vi "Select ini file.vi"(7 "error in":errorcluster) -> (0 "error out":errorcluster, 1 "Name":string)   [LabVIEW 2015]
uses:
  New Instance.ctl
  Instance.ctl
  Calibration and Function folders.ctl
  file/file action.ctl
  calibration/Shared Data/share data command.ctl
panel:
  in  "Delete Instance":bool
  in  "Device control":T1 {"Device" items=["Dev6", "Dev10", "Dev11"]}
  in  "Select":bool[](array[boolean])
  out "Instances":T2[](array[typedef])
  in  "New ProCoDA":T3
  in  "OK Button":bool
  # "Currently in use"
  # "Name of this instance"
  # "Method file name"
  # "Name of DAQ"
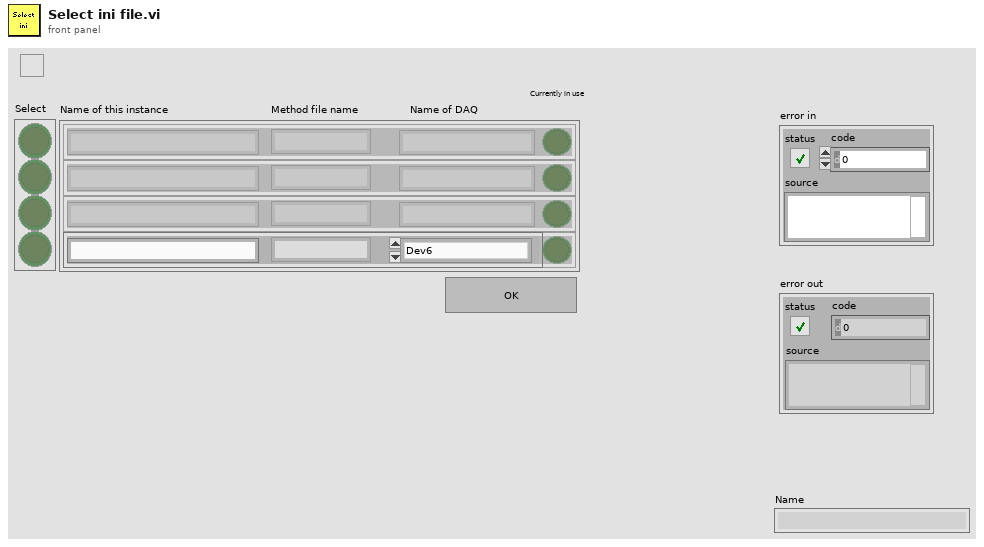
[diagram p1: front panel]
types:
  T1 = cluster{"Name":string, "File Name":string, "Device":u16}
  T2 = typedef "Instance.ctl" = cluster{"Name":string, "Device Name":string, "Running":bool, "File Name":string}
  T3 = typedef "New Instance.ctl" = bool
  T4 = typedef "Calibration and Function folders.ctl" = enum16{"Sensors", "Functions", "Config File", "PublicAppFolder", "New ini File", "Set Config File", "Delete ini File"}
  T5 = typedef "share data command.ctl" = enum16{"Initialize from ini", "Update ini", "Write data", "Read data", "List my data", "List shared data", "Close"}
  T6 = typedef "file action.ctl" = enum16{"Save", "Open"}
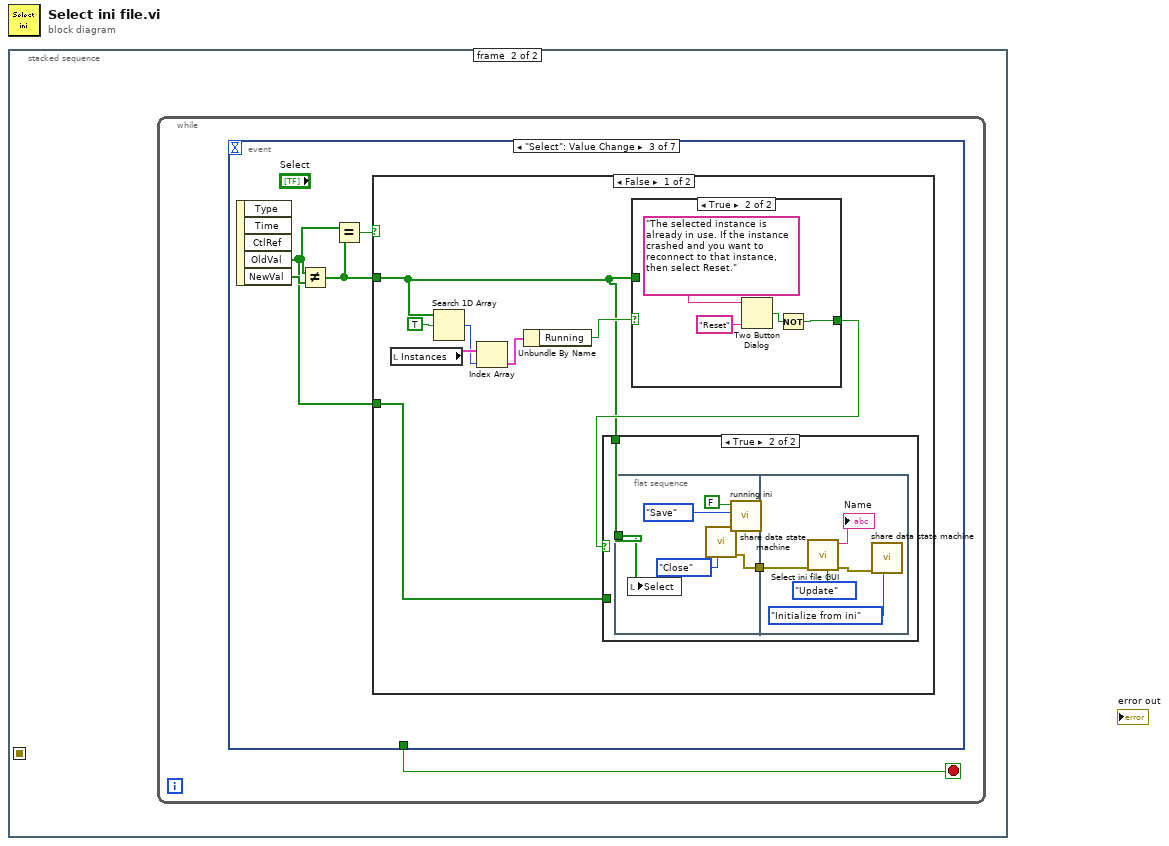
[diagram p0: block diagram]
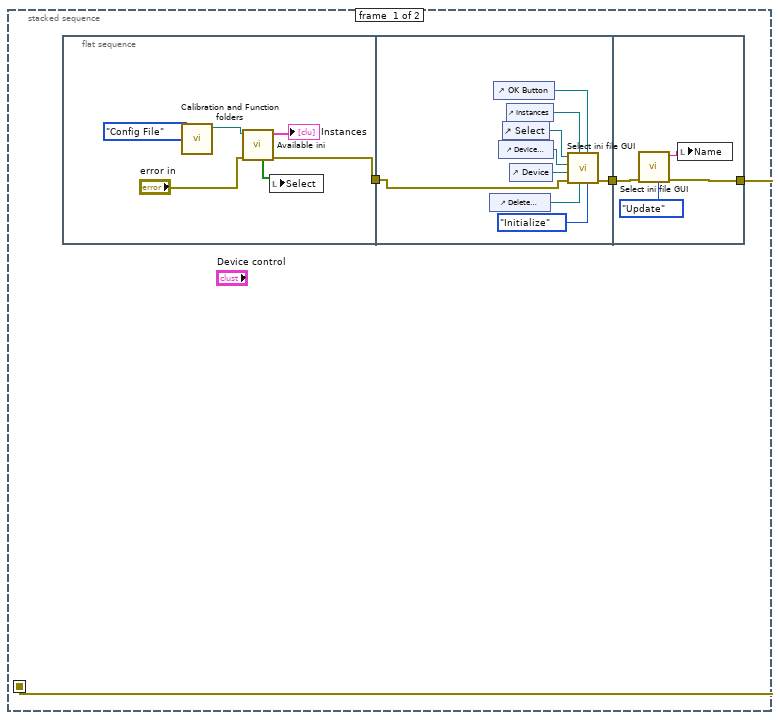
[diagram p2: hidden frame]
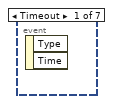
[diagram p3: hidden frame]
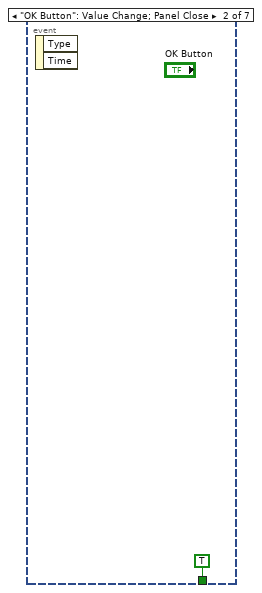
[diagram p4: hidden frame]
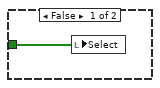
[diagram p5: hidden frame]
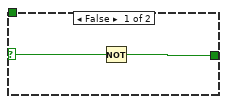
[diagram p6: hidden frame]
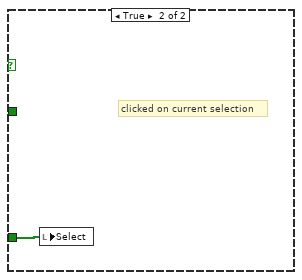
[diagram p7: hidden frame]
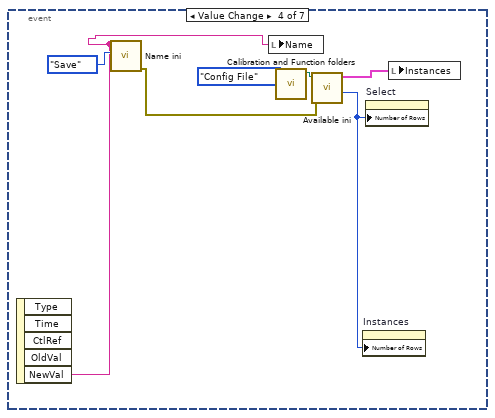
[diagram p8: hidden frame]
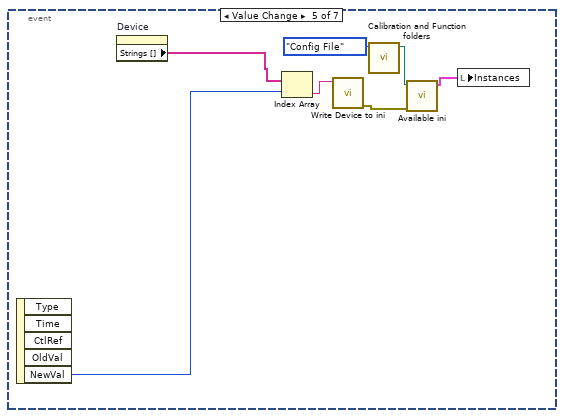
[diagram p9: hidden frame]
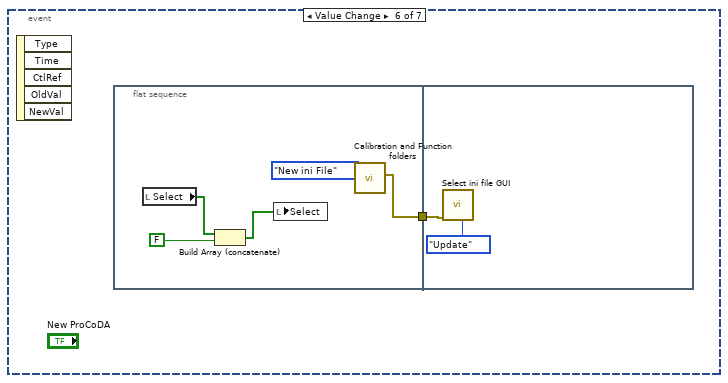
[diagram p10: hidden frame]
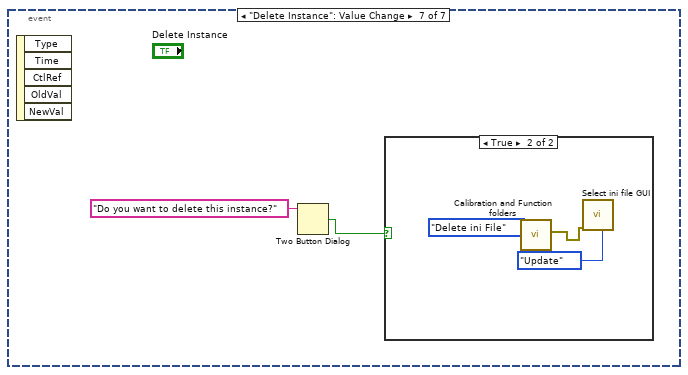
[diagram p11: hidden frame]
diagram:
  n1 = stacked-sequence {
    seq-local: [w2 _] -> [_ _]
    frame #0 {
      n2 = flat-sequence {
        tunnel: [w4] -> w3
        tunnel: w3 -> [w13]
        tunnel: [w12] -> w1
        tunnel: [w21] -> w2
        tunnel: w1 -> [w22]
        frame #0 {
          n3 = call "Calibration and Function folders.vi"("Folder"=Calibration_and_Function_folders."Config File") -> ("Selected Folder"=w9:path)  [unwired: 9 in, 1 out]
          n4 = call "Available ini.vi"("error in"="error in", "Config file path"=w9) -> ("error out"=w4:errorcluster, "Instances"=→"Instances":T2[], "Select"=w5:bool[])  [unwired: 4 in, 3 out]
          n5 = local write "Select"(w5) -> ()
        }
        frame #1 {
          n6 = control-ref of="Delete Instance"() -> (w14:refnum<vi>)
          n7 = control-ref of="OK Button"() -> (w10:refnum<vi>)
          n8 = control-ref of="Device control"() -> (w16:refnum<vi>)
          n9 = control-ref of="Select"() -> (w18:refnum<vi>)
          n10 = control-ref of="Instances"() -> (w17:refnum<vi>)
          n11 = control-ref of="Device"() -> (w15:refnum<vi>)
          n12 = call "Select ini file GUI.vi"("Command"=enum16{"Initialize", "Update"}."Initialize", "ok"=w10, "Delete Instance"=w14, "Instances"=w17, "error in (no error)"=w13, "Device"=w15, "Device control"=w16, "Select"=w18) -> ("error out"=w12:errorcluster)  [unwired: 2 in, 1 out]
        }
        frame #2 {
          n13 = call "Select ini file GUI.vi"("Command"=enum16{"Initialize", "Update"}."Update", "error in (no error)"=w22) -> ("error out"=w21:errorcluster, "Name"=w20:string)  [unwired: 8 in]
          n14 = local write "Name"(w20) -> ()
        }
      }
    }
    frame #1 {
      n15 = while {
        stop <- w23 stop-if-true
        n16 = event shown="[2] \"Select\": Value Change" {
          selector: _ -> [_ _ _ _ _ _ _]
          dyn-events: _ -> [_ _ _ _ _ _ _]
          timeout: _ -> [_ _ _ _ _ _ _]
          tunnel: [_ TRUE ("OK Button") _ _ _ _ _] -> w23
          event Timeout {
            n17 = event-data() -> ()  [unwired: 1 in, 2 out]
          }
          event "OK Button": Value Change; Panel Close {
            n18 = event-data() -> ()  [unwired: 1 in, 2 out]
          }
          event "Select": Value Change {
            n19 = event-data() -> ("OldVal"=w27:bool[], "NewVal"=w28:bool[])  [unwired: 1 in, 3 out]
            n20 = Not Equal?(x=w27, y=w28) -> (x != y?=w26:bool[])
            n21 = Equal?(x=w27, y=w26) -> (x = y?=w25:bool)
            n22 = case shown="False" w25 {
              tunnel: w27 -> [w30 w56]
              tunnel: w26 -> [w29 _]
              frame False {
                n23 = local read "Instances"() -> (w35:T2[])
                n24 = Search 1D Array(1D array=w29, element=TRUE) -> (index of element=w34:i32)  [unwired: 1 in]
                n25 = Index Array(array=w35, index=w34) -> (element=w33:T2)
                n26 = Unbundle By Name(w33) -> ("Running"=w32:bool)
                n27 = case shown="True" w32 {
                  selector: w32 -> [w51 _]
                  tunnel: w29 -> [_ _]
                  tunnel: [w50 w52] -> w31
                  frame False {
                    n28 = Not(x=w51) -> (.not. x?=w50:bool)
                  }
                  frame True {
                    n29 = Two Button Dialog(message="The selected instance is already in use. If the instance crashed and you want to reconnect to that instance, then select Reset.", 1:"Reset" ("F button name (\"Cancel\")")) -> (T button?=w53:bool)  [unwired: 1 in]
                    n30 = Not(x=w53) -> (.not. x?=w52:bool)
                  }
                }
                n31 = case shown="True" w31 {
                  tunnel: w29 -> [_ w39]
                  tunnel: w30 -> [w37 _]
                  frame False {
                    n32 = local write "Select"(w37) -> ()
                  }
                  frame True {
                    n33 = flat-sequence {
                      tunnel: w39 -> [w42]
                      tunnel: [w40] -> w38
                      tunnel: w38 -> [w47]
                      frame #0 {
                        n34 = local write "Select"(w42) -> ()
                        n35 = call "share data state machine.vi"("Share data command"=share_data_command."Close") -> ("error out"=w40:errorcluster)  [unwired: 4 in, 6 out]
                        n36 = call "running ini.vi"("running in"=FALSE ("running"), "Action"=file_action."Save") -> ()  [unwired: 4 in, 1 out]
                      }
                      frame #1 {
                        n37 = call "Select ini file GUI.vi"("Command"=enum16{"Initialize", "Update"}."Update", "error in (no error)"=w47) -> ("error out"=w45:errorcluster, "Name"=→"Name":string)  [unwired: 8 in]
                        n38 = call "share data state machine.vi"("Share data command"=share_data_command."Initialize from ini", "error in (no error)"=w45) -> ()  [unwired: 3 in, 7 out]
                      }
                    }
                  }
                }
              }
              frame True {
                # "clicked on current selection"
                n39 = local write "Select"(w56) -> ()
              }
            }
          }
          event "Device control.Name": Value Change {
            n40 = event-data() -> ("NewVal"=w57:string)  [unwired: 1 in, 4 out]
            n41 = call "Name ini.vi"("Action"=file_action."Save", "Name in"=w57) -> ("error out"=w58:errorcluster)  [unwired: 6 in, 1 out]
            n42 = local write "Name"(w57) -> ()
            n43 = call "Calibration and Function folders.vi"("Folder"=Calibration_and_Function_folders."Config File") -> ("Selected Folder"=w61:path)  [unwired: 9 in, 1 out]
            n44 = call "Available ini.vi"("error in"=w58, "Config file path"=w61) -> ("Size"=w62:i32, "Instances"=w59:T2[])  [unwired: 4 in, 4 out]
            n45 = property on="Instances" class="Arr (strict)"("Number of Rows"=w62) -> ()  [unwired: 2 in, 2 out]
            n46 = property on="Select" class="Arr (strict)"("Number of Rows"=w62) -> ()  [unwired: 2 in, 2 out]
            n47 = local write "Instances"(w59) -> ()
          }
          event "Device control.Device": Value Change {
            n48 = event-data() -> ("NewVal"=w65:u16)  [unwired: 1 in, 4 out]
            n49 = property on="Device" class="Ring (strict)"() -> ("Strings []"=w64:string[])  [unwired: 2 in, 2 out]
            n50 = Index Array(array=w64, index=w65) -> (element=w67:string)
            n51 = call "Write Device to ini.vi"("Device Name"=w67) -> ("error out"=w66:errorcluster)  [unwired: 10 in]
            n52 = call "Calibration and Function folders.vi"("Folder"=Calibration_and_Function_folders."Config File") -> ("Selected Folder"=w68:path)  [unwired: 9 in, 1 out]
            n53 = call "Available ini.vi"("error in"=w66, "Config file path"=w68) -> ("Instances"=w69:T2[])  [unwired: 4 in, 5 out]
            n54 = local write "Instances"(w69) -> ()
          }
          event Value Change {
            n55 = event-data() -> ()  [unwired: 1 in, 5 out]
            n56 = flat-sequence {
              tunnel: [w75] -> w71
              tunnel: w71 -> [w78]
              frame #0 {
                n57 = local read "Select"() -> (w74:bool[])
                n58 = Build Array (concatenate)(w74, FALSE) -> (w72:bool[])
                n59 = local write "Select"(w72) -> ()
                n60 = call "Calibration and Function folders.vi"("Folder"=Calibration_and_Function_folders."New ini File") -> ("error out"=w75:errorcluster)  [unwired: 9 in, 1 out]
              }
              frame #1 {
                n61 = call "Select ini file GUI.vi"("Command"=enum16{"Initialize", "Update"}."Update", "error in (no error)"=w78) -> ()  [unwired: 8 in, 2 out]
              }
            }
          }
          event "Delete Instance": Value Change {
            n62 = event-data() -> ()  [unwired: 1 in, 5 out]
            n63 = Two Button Dialog(message="Do you want to delete this instance?") -> (T button?=w79:bool)  [unwired: 2 in]
            n64 = case shown="True" w79 {
              frame False {
              }
              frame True {
                n65 = call "Calibration and Function folders.vi"("Folder"=Calibration_and_Function_folders."Delete ini File") -> ("error out"=w82:errorcluster)  [unwired: 9 in, 1 out]
                n66 = call "Select ini file GUI.vi"("Command"=enum16{"Initialize", "Update"}."Update", "error in (no error)"=w82) -> ()  [unwired: 8 in, 2 out]
              }
            }
          }
        }
      }
    }
  }
